vi "判断失败.vi"(1 "数组":i16[][](array[numeric])) -> (0 "布尔":bool)   [LabVIEW 2020]
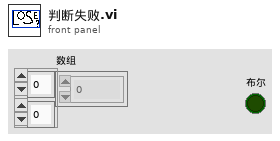
[diagram p1: front panel]
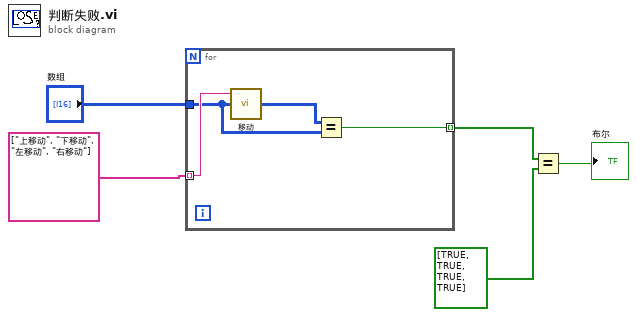
[diagram p0: block diagram]
diagram:
  n1 = for {
    tunnel: "数组" -> [w8]
    tunnel: string[] ["上移动", "下移动", "左移动", "右移动"] -> [w9] mode=indexing
    tunnel: [w6] -> w3 mode=indexing
    n2 = call "移动.vi"("移动前"=w8, "移动方式"=w9) -> ("移动后"=w7:i32[][])  [unwired: 1 in, 1 out]
    n3 = Equal?(x=w7, y=w8) -> (x = y?=w6:bool)
  }
  n4 = Equal?(x=w3, y=bool[] [TRUE, TRUE, TRUE, TRUE]) -> (x = y?=→"布尔":bool)
